vi "JSButtonsToString.vi"(8 "error in (no error)":errorcluster, 10 "Buttons":T1, 11 "JS ID":i32) -> (0 "error out":errorcluster, 3 "Button String":string)   [LabVIEW 2012]
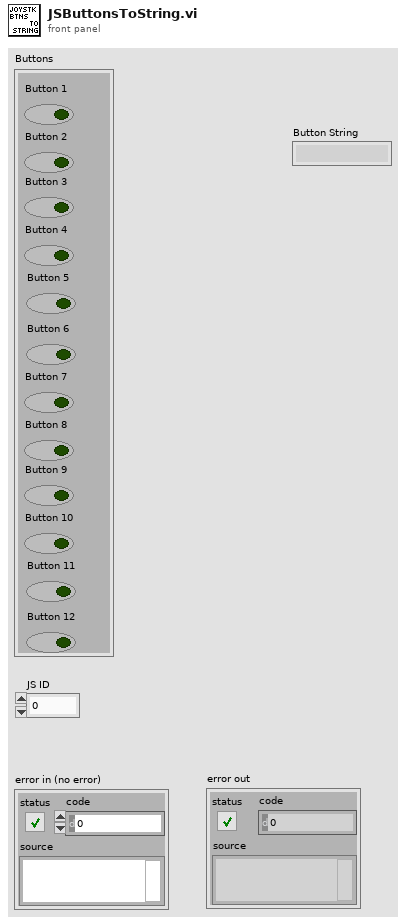
[diagram p1: front panel]
types:
  T1 = cluster{"Button 1":bool, "Button 2":bool, "Button 3":bool, "Button 4":bool, "Button 5":bool, "Button 6":bool, "Button 7":bool, "Button 8":bool, "Button 9":bool, "Button 10":bool, "Button 11":bool, "Button 12":bool}
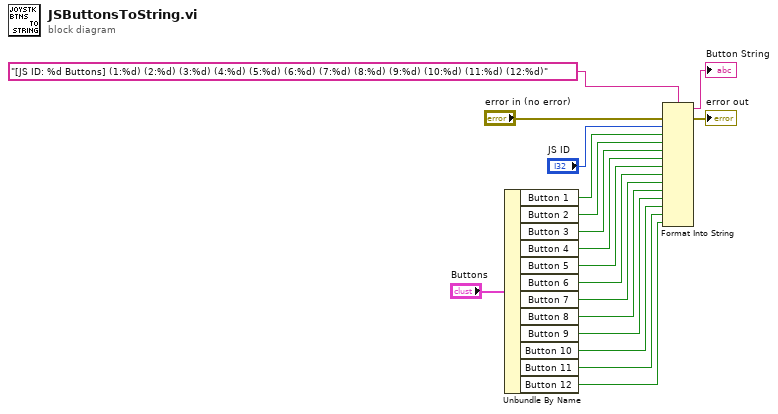
[diagram p0: block diagram]
diagram:
  n1 = Unbundle By Name("Buttons") -> ("Button 1"=w15:bool, "Button 2"=w14:bool, "Button 3"=w13:bool, "Button 4"=w12:bool, "Button 5"=w11:bool, "Button 6"=w10:bool, "Button 7"=w9:bool, "Button 8"=w8:bool, "Button 9"=w7:bool, "Button 10"=w6:bool, "Button 11"=w5:bool, "Button 12"=w4:bool)
  n2 = Format Into String(format string="[JS ID: %d Buttons] (1:%d) (2:%d) (3:%d) (4:%d) (5:%d) (6:%d) (7:%d) (8:%d) (9:%d) (10:%d) (11:%d) (12:%d)", error in="error in (no error)", "JS ID", w15, w14, w13, w12, w11, w10, w9, w8, w7, w6, w5, w4) -> (resulting string=→"Button String":string, error out=→"error out":errorcluster)  [unwired: 1 in]
